vi "TSM Relay Configuration Array Publish Desired State.vi"(0 "TSM Relay Configuration in":T1[](array[typedef]) {"SSC Relay with Action"."Relay Action" items=["Open Relay"=20, "Close Relay"=21]}, 1 "Published Data Id":string, 5 "index":i32, 7 "Completed Relay Operations":T4[](array[typedef]) {"Desired State" items=["Open Relay"=20, "Close Relay"=21]}, 11 "error in":errorcluster) -> (4 "TSM Relay Configuration out":T1[](array[typedef]) {"SSC Relay with Action"."Relay Action" items=["Open Relay"=20, "Close Relay"=21]}, 15 "error out":errorcluster)   [LabVIEW 2019]
doc: "This VI publishes the Desired State information from each Relay in the TSM Relay Configuration."
uses:
  SubVIs/TSM Relay Config.ctl
  <vilib>/NI_TestStand_SemiconductorModule/NI_TestStand_Semiconductor_Module.lvlibp/PinMap/PinQueryContext/MultiplePinMultipleSessionQueryContext/MultiplePinMultipleSessionQueryContext.lvclass
  C:/Program Files/National Instruments/LabVIEW 2019/vi.lib/NI_TestStand_SemiconductorModule/NI_TestStand_Semiconductor_Module.lvlibp/PinMap/PinQueryContext/MultipleSessionPinQueryContext.lvclass
  SSC/SSC Relay.ctl
  <instrlib>/niSwitch/niSwitch.llb/niSwitch Relay Action.ctl
  SubVIs/TSM Relay Completed Operations.ctl
  SubVIs/TSM Relay Per-Site to Per-Instrument Data.vi
  <vilib>/NI_TestStand_SemiconductorModule/NI_TestStand_Semiconductor_Module.lvlibp/PinMap/General/Publish/PublishDataWithContext.vi
  <vilib>/NI_TestStand_SemiconductorModule/NI_TestStand_Semiconductor_Module.lvlibp/PinMap/General/Publish/PublishDataDouble2D.vi
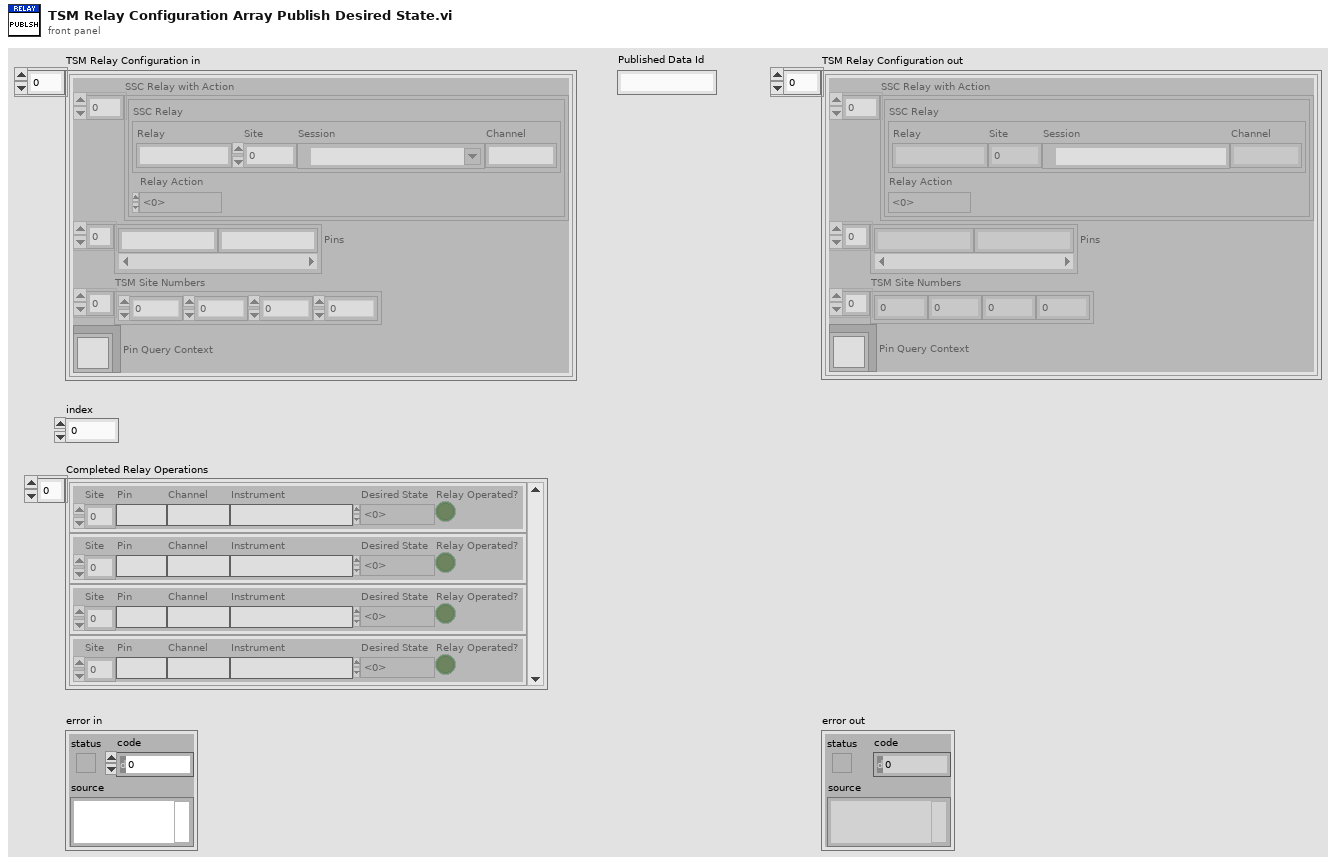
[diagram p1: front panel]
types:
  T1 = typedef "TSM Relay Config.ctl" = cluster{"SSC Relay with Action":cluster{"SSC Relay":T2, "Relay Action":T3}[], "Pins":string[], "TSM Site Numbers":i32[], "Pin Query Context":refnum<class "MultiplePinMultipleSessionQueryContext.lvclass">}
  T2 = typedef "SSC Relay.ctl" = cluster{"Relay":string, "Site":i32, "Session":refnum<k15>, "Channel":string}
  T3 = typedef "niSwitch Relay Action.ctl" = i32
  T4 = typedef "TSM Relay Completed Operations.ctl" = cluster{"Site":i32, "Pin":string, "Channel":string, "Instrument":string, "Desired State":T3, "Relay Operated?":bool}
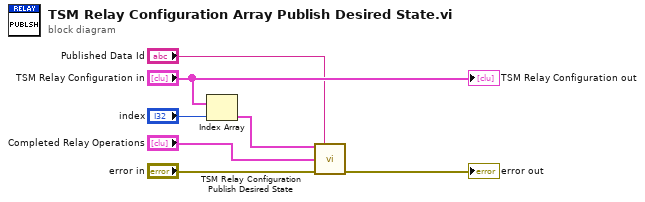
[diagram p0: block diagram]
diagram:
  n1 = Index Array(array="TSM Relay Configuration in", index="index") -> (element=w3:T1)
  n2 = call "TSM Relay Configuration Publish Desired State.vi"("TSM Relay Configuration in"=w3, "Published Data Id"="Published Data Id", "Completed Relay Operations"="Completed Relay Operations", "error in"="error in") -> ("error out"=→"error out":errorcluster)  [unwired: 10 in, 1 out]
  "TSM Relay Configuration out" <- "TSM Relay Configuration in"
